vi "dateSelect.vi"() -> ()   [LabVIEW 2012]
panel:
  in  "結束日期":refnum<k7>(container)
  out "From Date (起日)":string
  in  "請選開始日期":refnum<k7>(container)
  out "From Date (起日)":string
  in  "Shift (班別)":string(combo)
  in  "執行":bool
  in  "離開":bool
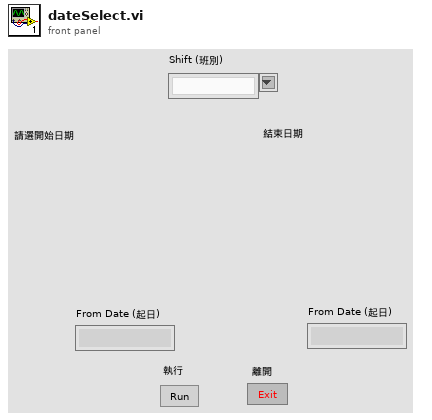
[diagram p1: front panel]
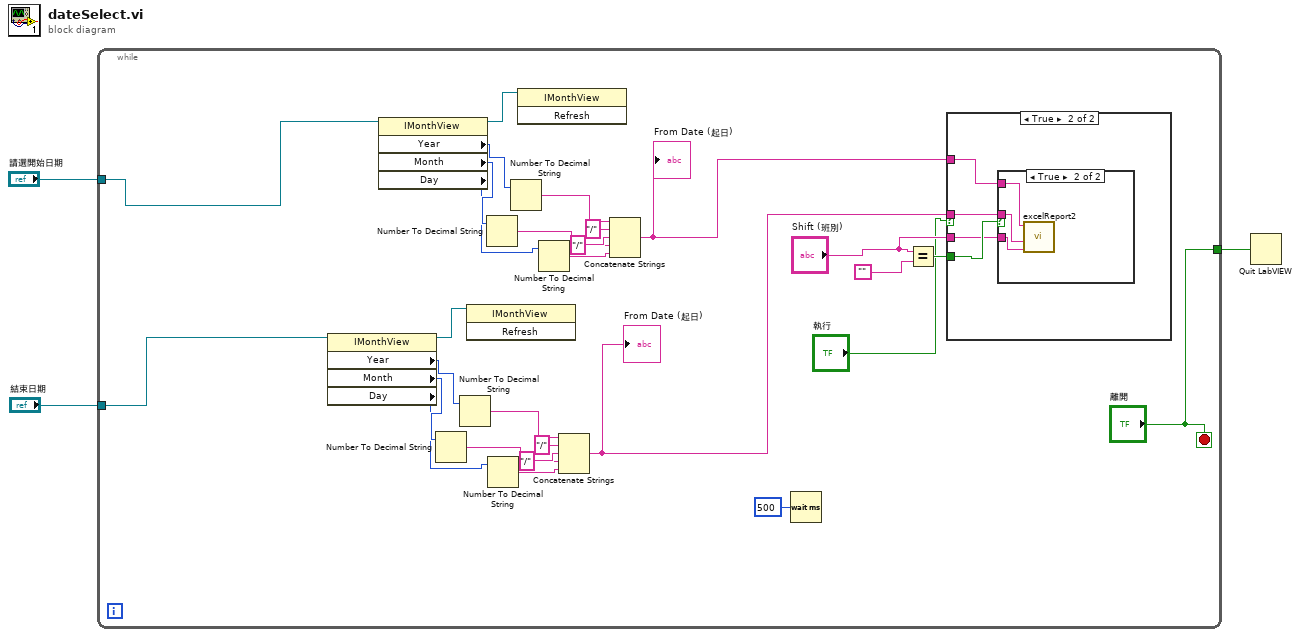
[diagram p0: block diagram]
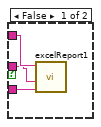
[diagram p3: hidden frame]
diagram:
  n1 = while {
    tunnel: ["離開"] -> w3
    tunnel: "請選開始日期" -> [w16]
    tunnel: "結束日期" -> [w6]
    stop <- "離開" stop-if-true
    n2 = property class="IMonthView"(reference=w6) -> (reference out=w15:refnum<k7>, "Year"=w14:i16, "Month"=w13:i32, "Day"=w12:i16)  [unwired: 1 in, 1 out]
    n3 = property class="IMonthView"(reference=w16) -> (reference out=w26:refnum<k7>, "Year"=w25:i16, "Month"=w24:i32, "Day"=w23:i16)  [unwired: 1 in, 1 out]
    n4 = Number To Decimal String(number=w13) -> (decimal integer string=w9:string)  [unwired: 1 in]
    n5 = Number To Decimal String(number=w14) -> (decimal integer string=w11:string)  [unwired: 1 in]
    n6 = invoke class="IMonthView" method="Refresh"(reference=w15) -> ()  [unwired: 2 in, 3 out]
    n7 = Number To Decimal String(number=w24) -> (decimal integer string=w20:string)  [unwired: 1 in]
    n8 = Number To Decimal String(number=w12) -> (decimal integer string=w7:string)  [unwired: 1 in]
    n9 = Number To Decimal String(number=w25) -> (decimal integer string=w22:string)  [unwired: 1 in]
    n10 = invoke class="IMonthView" method="Refresh"(reference=w26) -> ()  [unwired: 2 in, 3 out]
    n11 = Number To Decimal String(number=w23) -> (decimal integer string=w18:string)  [unwired: 1 in]
    n12 = Concatenate Strings(w11, "/" ("string"), w9, "/" ("string"), w7) -> (w5:string)
    "From Date (起日)" <- w5
    n13 = Concatenate Strings(w22, "/" ("string"), w20, "/" ("string"), w18) -> (w17:string)
    "From Date (起日)" <- w17
    n14 = Wait (ms)(milliseconds to wait=u32 500) -> ()  [unwired: 1 out]
    n15 = Equal?(x="Shift (班別)", y="") -> (x = y?=w30:bool)
    n16 = case shown="True" "執行" {
      tunnel: w30 -> [_ w35]
      tunnel: w5 -> [_ w34]
      tunnel: "Shift (班別)" -> [_ w33]
      tunnel: w17 -> [_ w32]
      frame False {
      }
      frame True {
        n17 = case shown="True" w35 {
          tunnel: w32 -> [w38 w41]
          tunnel: w34 -> [w37 w40]
          tunnel: w33 -> [w36 w39]
          frame False {
            n18 = call "excelReport1.vi"("Shift"=w36, "End Date"=w37, "From Date"=w38) -> ()  [unwired: 9 in]
          }
          frame True {
            n19 = call "excelReport2.vi"("Shift"=w39, "End Date"=w40, "From Date"=w41) -> ()  [unwired: 9 in]
          }
        }
      }
    }
  }
  n20 = Quit LabVIEW(quit? (T)=w3) -> ()
